vi "Wojtyna_Host_C.vi"() -> ()   [LabVIEW 2020]
panel:
  out "Waveform Graph":dbl[](graph)
  in  "SignalSend":bool
  in  "Stop":bool
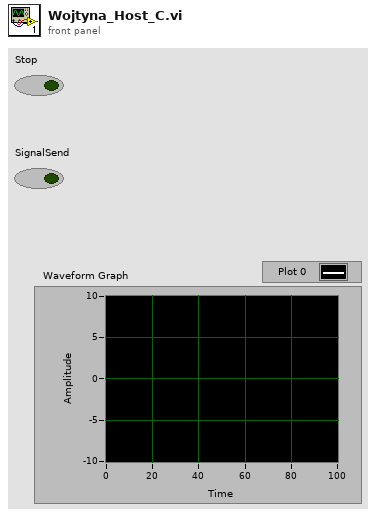
[diagram p1: front panel]
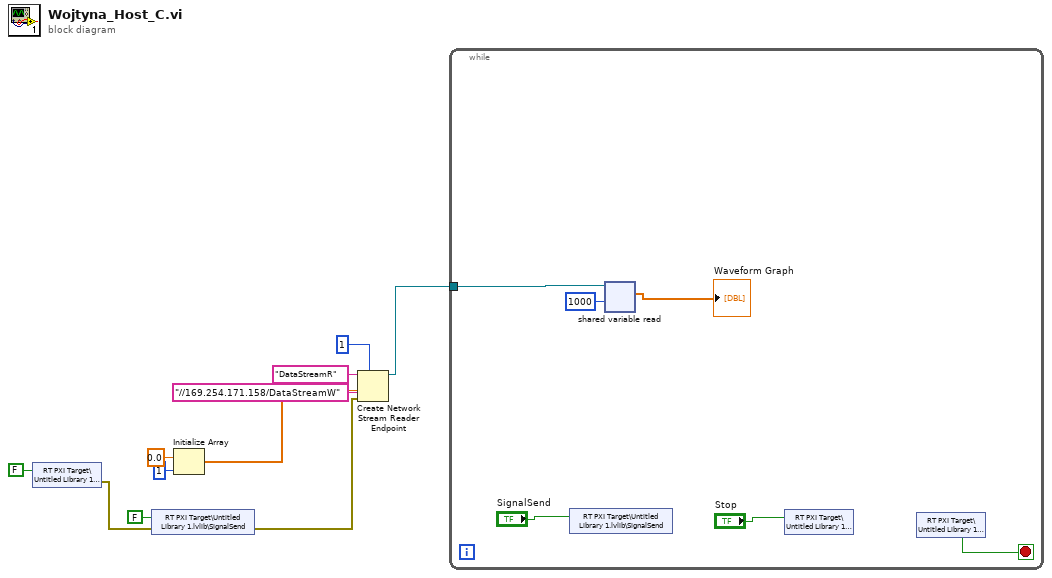
[diagram p0: block diagram]
diagram:
  n1 = shared-variable "RT PXI Target\\Untitled Library 1.lvlib\\Stop"(FALSE ("Stop")) -> (error out=w7:errorcluster)  [unwired: 1 in]
  n2 = shared-variable "RT PXI Target\\Untitled Library 1.lvlib\\SignalSend"(FALSE ("SignalSend"), error in=w7) -> (error out=w5:errorcluster)
  n3 = Initialize Array(0.0 ("element"), 1 ("dimension size")) -> (w1:dbl[])
  n4 = Create Network Stream Reader Endpoint(7:1 ("reader buffer size"), 8:w5, 9:w1, 10:"//169.254.171.158/DataStreamW" ("writer url"), 11:"DataStreamR" ("reader name")) -> (3:w4:refnum<k21>)  [unwired: 2 in, 1 out]
  n5 = while {
    tunnel: w4 -> [w14]
    stop <- w16 stop-if-true
    n6 = shared-variable "RT PXI Target\\Untitled Library 1.lvlib\\SignalSend"("SignalSend") -> ()  [unwired: 1 in, 1 out]
    n7 = shared-variable-read(w14, 1000 ("timeout ms (-1)")) -> (→"Waveform Graph":dbl[])  [unwired: 1 in, 3 out]
    n8 = shared-variable "RT PXI Target\\Untitled Library 1.lvlib\\Stop"("Stop") -> ()  [unwired: 1 in, 1 out]
    n9 = shared-variable "RT PXI Target\\Untitled Library 1.lvlib\\Stop"() -> (w16:bool)  [unwired: 1 in, 1 out]
  }
